vi "svfa_Initial Guess for Tone Estimation (complex).vi"(8 "FFT size":i32, 9 "window size":i32, 10 "window":T1(ring), 11 "three fingers":cluster{"f0":dbl, "df":dbl, "spectrum":cdb[]}={"f0"=0.0, "df"=1.0, "spectrum"=[]} {"spectrum" format="%.2f"; "df" format="%.4f"; "f0" format="%.5f"}) -> (0 "range":cluster{"f upper":dbl, "f lower":dbl} {"f lower" format="%.5f"; "f upper" format="%.5f"}, 3 "initial guess":dbl format="%.9f")   [LabVIEW 2017]
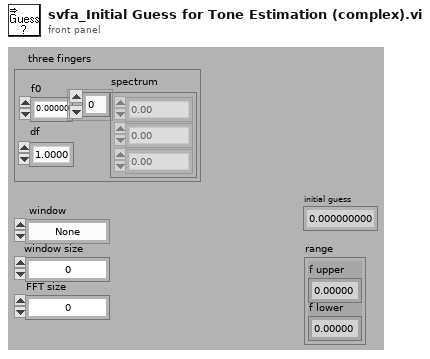
[diagram p1: front panel]
types:
  T1 = enum16{"None ", "Hanning", "Hamming", "Blackman-Harris", "Exact Blackman", "Blackman", "Flat Top", "4 Term B-Harris ", "7 Term B-Harris", "Low Sidelobe"}
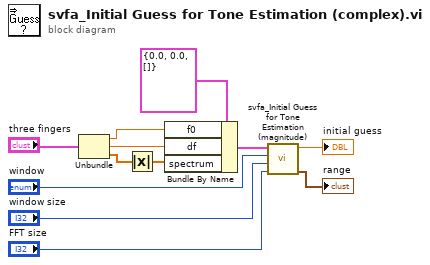
[diagram p0: block diagram]
diagram:
  n1 = Unbundle("three fingers") -> ("f0"=w11:dbl, "df"=w10:dbl, "spectrum"=w9:cdb[])
  n2 = Absolute Value(x=w9) -> (abs(x)=w7:dbl[])
  n3 = Bundle By Name(cluster=cluster{"f0":dbl, "df":dbl, "spectrum":dbl[]} {"f0"=0.0, "df"=0.0, "spectrum"=[]} ("three fingers 2"), "f0"=w11, "df"=w10, "spectrum"=w7) -> (w8:cluster{"f0":dbl, "df":dbl, "spectrum":dbl[]})
  n4 = call <vilib>:"svfa_Initial Guess for Tone Estimation (magnitude).vi"("FFT size"="FFT size", "window size"="window size", "window"="window", "three fingers"=w8) -> ("range"=→"range":cluster{"f upper":dbl, "f lower":dbl}, "initial guess"=→"initial guess":dbl)  [unwired: 6 in]
